vi "pInitialize.vi"(8 "error in":errorcluster, 9 "Internal":string[](array[string]), 10 "Inputs in":string[](array[string]), 11 "Output":string[](array[string])) -> (0 "error out":errorcluster, 2 "data dictionary out":refnum<class "data dictionary.lvclass">, 3 "default data table":T1, 4 "Outputs":string[](array[string])=["A", "A+", "A-", "B", "B+", "B-", "S1", "S2", "S3", "S4", "S5", "S6", "S7"], 5 "Input Index":i32[](array[numeric]), 6 "Inputs out":string[](array[string])=["A", "A+", "A-", "B", "B+", "B-", "S1", "S2", "S3", "S4", "S5", "S6", "S7"], 7 "Output Index":i32[](array[numeric]))   [LabVIEW 2013]
uses:
  <vilib>/NI/Tag Bus/table/data table.ctl
  <vilib>/NI/Tag Bus/dictionary/data dictionary.lvclass
  <vilib>/NI/Tag Bus/tag/Data Type.ctl
  <vilib>/NI/Tag Bus/tag/tag descriptor.lvclass/tag descriptor.ctl
  <vilib>/NI/Tag Bus/dictionary/data dictionary.lvclass/data dictionary.ctl
  <vilib>/NI/Tag Bus/tag bus error generator.vi
  <vilib>/NI/Tag Bus/tag/validate default value.vi
  <vilib>/NI/Tag Bus/tag/tag descriptor.lvclass
  <vilib>/NI/Tag Bus/table/data table.lvlib
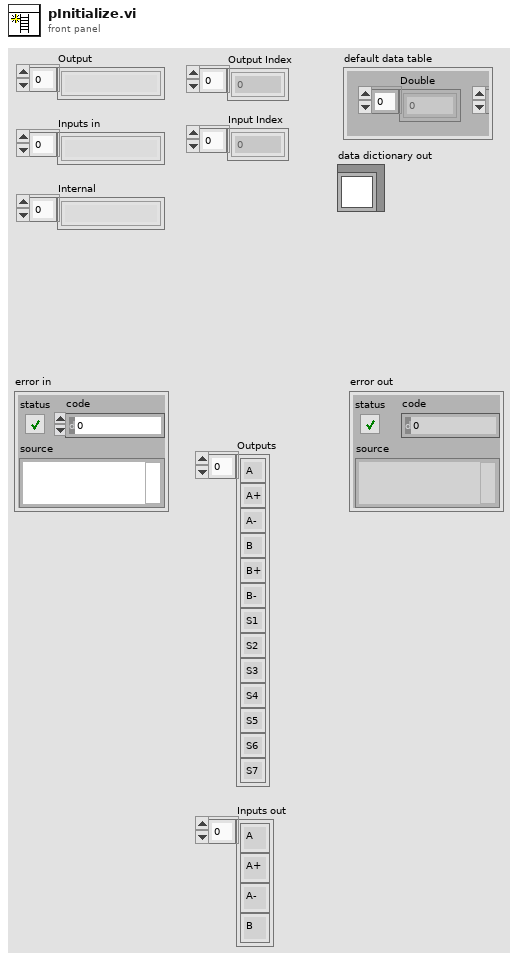
[diagram p1: front panel]
types:
  T1 = typedef "tag bus.lvlib/data table.lvlib/data table.ctl" = cluster{"Double":dbl[], "Single":sgl[], "I64":i64[], "I32":i32[], "I16":i16[], "I8":i8[], "U64":u64[], "U32":u32[], "U16":u16[], "U8":u8[], "Boolean":bool[], "String":string[], "Array of Double":cluster{"DBL Array":dbl[]}[], "Array of Single":cluster{"SGL Array":sgl[]}[], "Array of I64":cluster{"I64 Array":i64[]}[], "Array of I32":cluster{"I32 Array":i32[]}[], "Array of I16":cluster{"I16 Array":i16[]}[], "Array of I8":cluster{"I8 Array":i8[]}[], "Array of U64":cluster{"U64 Array":u64[]}[], "Array of U32":cluster{"U32 Array":u32[]}[], "Array of U16":cluster{"U16 Array":u16[]}[], "Array of U8":cluster{"U8 Array":u8[]}[], "Array of Boolean":cluster{"Boolean Array":bool[]}[], "Array of String":cluster{"String Array":string[]}[]}
  T2 = typedef "tag bus.lvlib/tag descriptor.lvclass/Data Type.ctl" = enum16{"Double", "Single", "I64", "I32", "I16", "I8", "U64", "U32", "U16", "U8", "Boolean", "String", "Array of Double", "Array of Single", "Array of I64", "Array of I32", "Array of I16", "Array of I8", "Array of U64", "Array of U32", "Array of U16", "Array of U8", "Array of Boolean", "Array of String"}
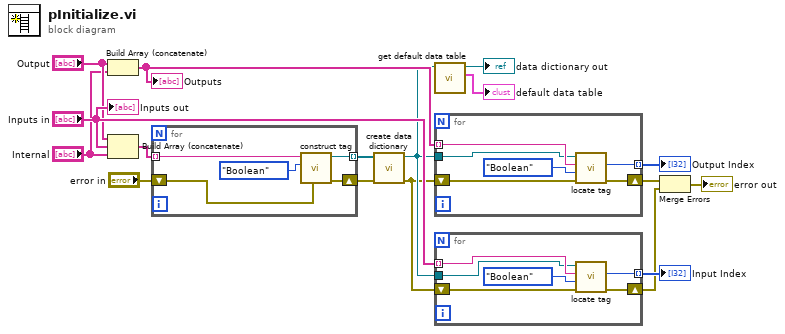
[diagram p0: block diagram]
diagram:
  n1 = Build Array (concatenate)("Output", "Internal") -> (w15:string[])
  "Outputs" <- w15
  n2 = Build Array (concatenate)("Output", "Inputs in", "Internal") -> (w10:string[])
  n3 = for {
    tunnel: [w22] -> w7 mode=indexing
    tunnel: w10 -> [w21] mode=indexing
    shift-right: [w18] -> w2
    shift-left: "error in" -> [w19]
    n4 = call <vilib>:"construct tag.vi"("error in"=w19, "data type"=Data_Type."Boolean", "name"=w21) -> ("error out"=w18:errorcluster, "system tag out"=w22:refnum<class "tag descriptor.lvclass">)  [unwired: 7 in]
  }
  n5 = call <vilib>:"create data dictionary.vi"("error in"=w2, "system tags"=w7) -> ("error out"=w1:errorcluster, "data dictionary"=w13:refnum<class "data dictionary.lvclass">)  [unwired: 8 in]
  n6 = call <vilib>:"get default data table.vi"("data dictionary in"=w13) -> ("default data table"=→"default data table":T1, "data dictionary out"=→"data dictionary out":refnum<class "data dictionary.lvclass">)  [unwired: 9 in]
  n7 = for {
    tunnel: w15 -> [w27] mode=indexing
    tunnel: w13 -> [w26]
    tunnel: [w25] -> w12 mode=indexing
    shift-right: [w24] -> w4
    shift-left: w1 -> [w23]
    n8 = call <vilib>:"locate tag.vi"("error in"=w23, "data type"=Data_Type."Boolean", "name"=w27, "data dictionary in"=w26) -> ("error out"=w24:errorcluster, "index"=w25:i32)  [unwired: 5 in, 1 out]
  }
  "Output Index" <- w12
  n9 = for {
    tunnel: "Inputs in" -> [w33] mode=indexing
    tunnel: w13 -> [w32]
    tunnel: [w31] -> w14 mode=indexing
    shift-right: [w30] -> w5
    shift-left: w1 -> [w29]
    n10 = call <vilib>:"locate tag.vi"("error in"=w29, "data type"=Data_Type."Boolean", "name"=w33, "data dictionary in"=w32) -> ("error out"=w30:errorcluster, "index"=w31:i32)  [unwired: 5 in, 1 out]
  }
  "Input Index" <- w14
  n11 = Merge Errors(w4, w5) -> (→"error out":errorcluster)
  "Inputs out" <- "Inputs in"
